vi "FlatToRichrfcontrol_GetRFTileSampleRateResponse.vi"(5 "OutputClusterType":T1, 11 "InputCluster":T2) -> (3 "OutputCluster":T1)   [LabVIEW 2024, in "FlexSDR_gRPC_client.lvlib"]
uses:
  FlexSDR_gRPC_client.lvlib
  rfcontrol_GetRFTileSampleRateResponse_Flat.ctl
  rfcontrol_GetRFTileSampleRateResponse.ctl
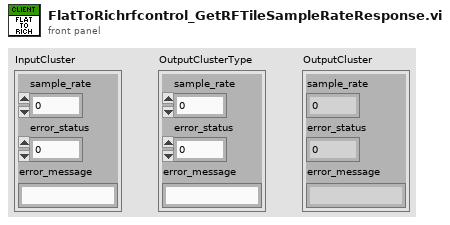
[diagram p1: front panel]
types:
  T1 = typedef "FlexSDR_gRPC_client.lvlib/rfcontrol_GetRFTileSampleRateResponse.ctl" = cluster{"sample_rate":dbl, "error_status":i32, "error_message":string}
  T2 = typedef "FlexSDR_gRPC_client.lvlib/rfcontrol_GetRFTileSampleRateResponse_Flat.ctl" = cluster{"sample_rate":dbl, "error_status":i32, "error_message":string}
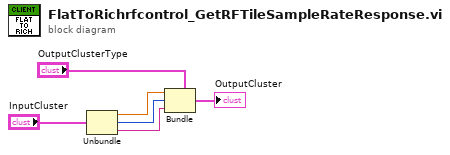
[diagram p0: block diagram]
diagram:
  n1 = Unbundle "Unbundle"("InputCluster") -> ("sample_rate"=w3:dbl, "error_status"=w2:i32, "error_message"=w1:string)
  n2 = Bundle "Bundle"(cluster="OutputClusterType", "sample_rate"=w3, "error_status"=w2, "error_message"=w1) -> (→"OutputCluster":T1)
